vi "PKG_IMC_LinePos.vi"(4 "fifo":i32, 5 "wait":i32, 6 "endvel":dbl, 7 "tgvel":dbl, 9 "axisNum":i32, 10 "pos":i32[](array[numeric])=array[4097 elements], 11 "handle":u32) -> (1 "function return":i32, 2 "pos out":i32[](array[numeric]), 3 "handle out":u32)   [LabVIEW 2011, in "IMC_Pkg4xxx.lvlib"]
doc: "PKG_IMC_Line_Pos(IMC_HANDLE handle, long pos[], int axisNum, double tgvel, double endvel, int wait, int fifo);"
uses:
  IMC_Pkg4xxx.lvlib
  IMC_Pkg4xxx.dll
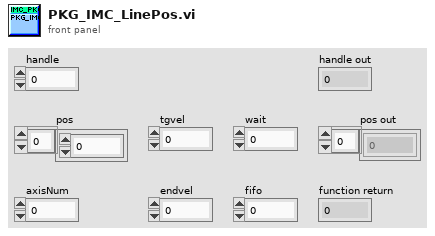
[diagram p1: front panel]
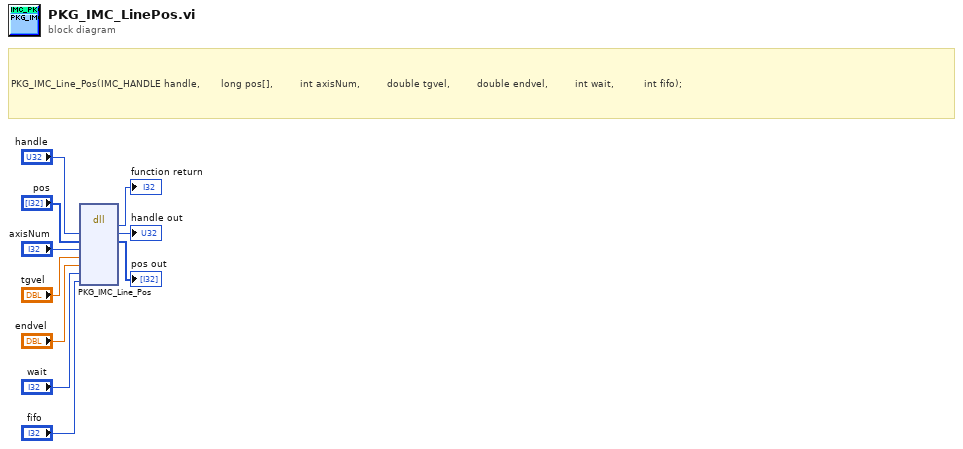
[diagram p0: block diagram]
diagram:
  # "PKG_IMC_Line_Pos(IMC_HANDLE handle, \t\t\t\t\t\tlong pos[], \t\t\t\t\t\t\t\tint axisNum, \t\t\t\t\t\t\t\tdouble tgvel, \t\t\t\t\t\t\t\tdouble endvel, \t\t\t\t\t\t\t\tint wait, \t\t\t\t\t\t\t\t\tint fifo);"
  n1 = dll-call lib="PTH1mabs F光盘刻录\niMC MotionIMCNet_V4.0IMCAppincLabviewIMC_PKG4xxxIMC_PKG4xxx\nIMC_Pkg4xxx.*" fn="PKG_IMC_Line_Pos"("handle"="handle", "pos"="pos", "axisNum"="axisNum", "tgvel"="tgvel", "endvel"="endvel", "wait"="wait", "fifo"="fifo") -> (→"function return":i32, "handle"=→"handle out":u32, "pos"=→"pos out":i32[])  [unwired: 8 in, 2 out]
